vi "Update Slots.vi"(6 "FPGA Target":T1, 8 "error in (no error)":errorcluster, 10 "Scan Mode Slots":u32[](array[numeric]), 11 "Item Ref in":T2 format="%.0x") -> (0 "error out":errorcluster, 3 "Item Ref out":T2 format="%.0x")   [LabVIEW 2016, in "Scan Engine Custom Device.lvlib"]
uses:
  Scan Engine Custom Device.lvlib
  <vilib>/NI Veristand/Custom Device API/Custom Device API.lvlib
  Globals/Scan Engine GUIDs.vi
  Modules.lvlibp/RSI Module/Module Models.ctl
  <vilib>/NI Veristand/Custom Device API/Custom Device Item Ref.ctl
  Type Defs/FPGA Target.ctl
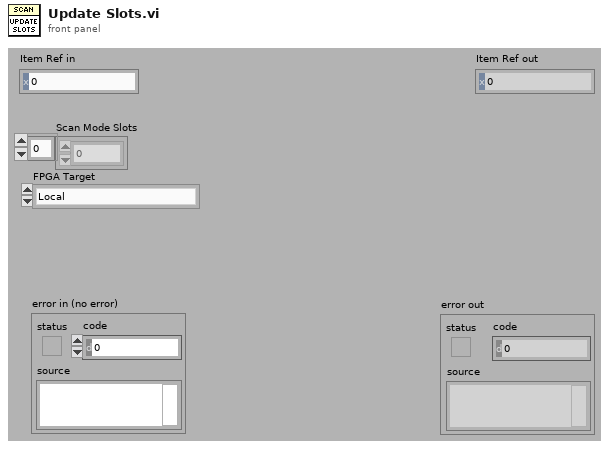
[diagram p1: front panel]
types:
  T1 = typedef "Scan Engine Custom Device.lvlib/FPGA Target.ctl" = enum16{"Local", "EtherCAT"}
  T2 = typedef "Custom Device API.lvlib/Custom Device Item Ref.ctl" = u64
  T3 = typedef "Modules.lvlibp/RSI Module.lvclass/Module Models.ctl" = enum16{"Empty", "NI 9201", "NI 9203", "NI 9205", "NI 9206", "NI 9207", "NI 9208", "NI 9211", "NI 9213", "NI 9214", "NI 9215", "NI 9217", "NI 9219", "NI 9221", "NI 9225", "NI 9227", "NI 9229", "NI 9233", "NI 9234", "NI 9235", "NI 9236", "NI 9237", "NI 9239", "NI 9263", "NI 9264", "NI 9265", "NI 9269", "NI 9375", "NI 9401", "NI 9402", "NI 9403", "NI 9411", "NI 9421", "NI 9422", "NI 9423", "NI 9425", "NI 9426", "NI 9435", "NI 9472", "NI 9474", "NI 9475", "NI 9476", "NI 9477", "NI 9478", "NI 9481", "NI 9482", "NI 9485"}
  T4 = typedef "Modules.lvlibp/Custom Device API.lvlib/Custom Device Item Ref.ctl" = u64
  T5 = typedef "Modules.lvlibp/RSI Module.lvclass/Slot Settings.ctl" = cluster{"Slot":u32, "EtherCAT?":bool}
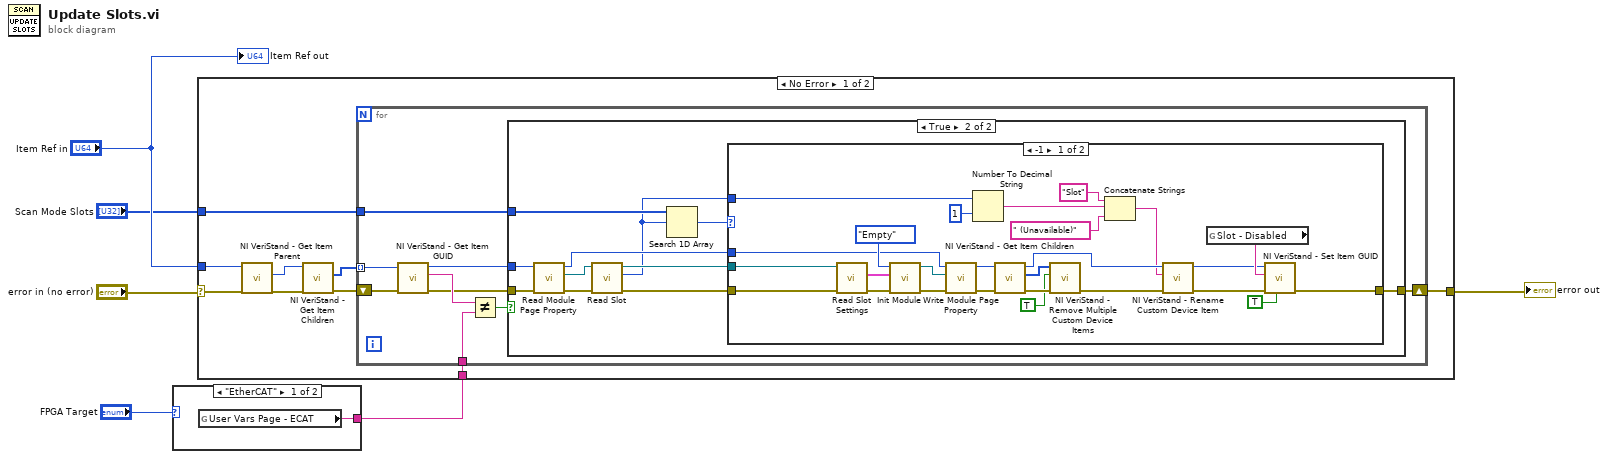
[diagram p0: block diagram]
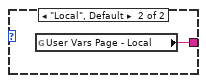
[diagram p2: hidden frame]
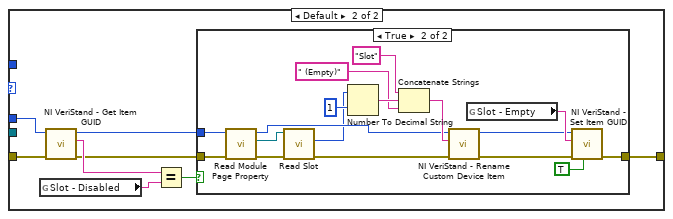
[diagram p4: hidden frame]
diagram:
  n1 = case shown="\"EtherCAT\"" "FPGA Target" {
    tunnel: [w7 w8] -> w1
    frame "EtherCAT" {
      n2 = global read "Scan Engine GUIDs.vi" "User Vars Page - ECAT"() -> (w7:string)
    }
    frame "Local", Default {
      n3 = global read "Scan Engine GUIDs.vi" "User Vars Page - Local"() -> (w8:string)
    }
  }
  n4 = case shown="No Error" "error in (no error)" {
    selector: "error in (no error)" -> [w16 w91]
    tunnel: [w9 w91] -> w5
    tunnel: "Item Ref in" -> [w17 _]
    tunnel: "Scan Mode Slots" -> [w11 _]
    tunnel: w1 -> [w10 _]
    frame No Error {
      n5 = call <vilib>:"NI VeriStand - Get Item Parent.vi"("error in (no error)"=w16, "Item Ref in"=w17) -> ("error out"=w15:errorcluster, "Parent Ref"=w14:T2)  [unwired: 6 in, 2 out]
      n6 = call <vilib>:"NI VeriStand - Get Item Children.vi"("error in (no error)"=w15, "Item Ref in"=w14) -> ("error out"=w13:errorcluster, "Child Refs"=w12:T2[])  [unwired: 6 in, 2 out]
      n7 = for {
        shift-right: [w18] -> w9
        shift-left: w13 -> [w26]
        tunnel: w12 -> [w25] mode=indexing
        tunnel: w11 -> [w19]
        tunnel: w10 -> [w24]
        n8 = call <vilib>:"NI VeriStand - Get Item GUID.vi"("error in (no error)"=w26, "Item Ref in"=w25) -> ("error out"=w21:errorcluster, "GUID"=w23:string, "Item Ref out"=w20:T2)  [unwired: 7 in]
        n9 = Not Equal?(x=w23, y=w24) -> (x != y?=w22:bool)
        n10 = case shown="True" w22 {
          tunnel: w21 -> [w27 w38]
          tunnel: w20 -> [_ w37]
          tunnel: w19 -> [_ w34]
          tunnel: [w27 w29] -> w18
          frame False {
          }
          frame True {
            n11 = call "Read Module Page Property.vi"("error in (no error)"=w38, "Node Ptr In"=w37) -> ("error out"=w36:errorcluster, "RSI Module"=w35:refnum<class "RSI Module.lvclass">, "Node Ptr Out"=w31:T4)  [unwired: 7 in]
            n12 = call "Read Slot.vi"("error in (no error)"=w36, "RSI Module in"=w35) -> ("error out"=w32:errorcluster, "Slot"=w28:u32, "RSI Module out"=w30:refnum<class "RSI Module.lvclass">)  [unwired: 7 in]
            n13 = Search 1D Array(1D array=w34, element=w28) -> (index of element=w33:i32)  [unwired: 1 in]
            n14 = case shown="-1" w33 {
              tunnel: w32 -> [w62 w67]
              tunnel: w31 -> [w56 w66]
              tunnel: w30 -> [w61 _]
              tunnel: [w49 w65] -> w29
              tunnel: w28 -> [w46 _]
              frame -1 {
                n15 = call "Read Slot Settings.vi"("error in (no error)"=w62, "RSI Module in"=w61) -> ("error out"=w60:errorcluster, "Slot Settings"=w59:T5)  [unwired: 7 in, 1 out]
                n16 = call "Init Module.vi"("error in (no error)"=w60, "Slot Settings"=w59, "Module Model"=Module_Models."Empty") -> ("error out"=w57:errorcluster, "RSI Module out"=w55:refnum<class "RSI Module.lvclass">)  [unwired: 7 in]
                n17 = call "Write Module Page Property.vi"("error in (no error)"=w57, "RSI Module"=w55, "Node Ptr In"=w56) -> ("error out"=w51:errorcluster, "Node Ptr Out"=w50:T4)  [unwired: 6 in, 1 out]
                n18 = Number To Decimal String(number=w46, width (-)=i16 1) -> (decimal integer string=w45:string)
                n19 = call <vilib>:"NI VeriStand - Get Item Children.vi"("error in (no error)"=w51, "Item Ref in"=w50) -> ("error out"=w54:errorcluster, "Child Refs"=w53:T2[], "Item Ref out"=w42:T2)  [unwired: 6 in, 1 out]
                n20 = call <vilib>:"NI VeriStand - Remove Multiple Custom Device Items.vi"("error in (no error)"=w54, "Force Delete (F)"=TRUE, "Item Refs in"=w53) -> ("error out"=w43:errorcluster)  [unwired: 7 in, 1 out]
                n21 = Concatenate Strings("Slot" ("string"), w45, " (Unavailable)" ("Section Name")) -> (w39:string)
                n22 = call <vilib>:"NI VeriStand - Rename Custom Device Item.vi"("error in (no error)"=w43, "New Name"=w39, "Item Ref in"=w42) -> ("error out"=w40:errorcluster, "Item Ref out"=w41:T2)  [unwired: 1 in, 6 out]
                n23 = global read "Scan Engine GUIDs.vi" "Slot - Disabled"() -> (w64:string)
                n24 = call <vilib>:"NI VeriStand - Set Item GUID.vi"("Refresh System Explorer Tree? (F)"=TRUE, "error in (no error)"=w40, "GUID"=w64, "Item Ref in"=w41) -> ("error out"=w49:errorcluster)  [unwired: 6 in, 1 out]
              }
              frame Default {
                n25 = global read "Scan Engine GUIDs.vi" "Slot - Disabled"() -> (w71:string)
                n26 = call <vilib>:"NI VeriStand - Get Item GUID.vi"("error in (no error)"=w67, "Item Ref in"=w66) -> ("error out"=w69:errorcluster, "GUID"=w72:string, "Item Ref out"=w68:T2)  [unwired: 7 in]
                n27 = Equal?(x=w72, y=w71) -> (x = y?=w70:bool)
                n28 = case shown="True" w70 {
                  tunnel: w69 -> [w73 w82]
                  tunnel: w68 -> [_ w83]
                  tunnel: [w73 w88] -> w65
                  frame False {
                  }
                  frame True {
                    n29 = call "Read Module Page Property.vi"("error in (no error)"=w82, "Node Ptr In"=w83) -> ("error out"=w85:errorcluster, "RSI Module"=w84:refnum<class "RSI Module.lvclass">, "Node Ptr Out"=w76:T4)  [unwired: 7 in]
                    n30 = call "Read Slot.vi"("error in (no error)"=w85, "RSI Module in"=w84) -> ("error out"=w74:errorcluster, "Slot"=w75:u32)  [unwired: 7 in, 1 out]
                    n31 = Number To Decimal String(number=w75, width (-)=i16 1) -> (decimal integer string=w80:string)
                    n32 = Concatenate Strings("Slot" ("string"), w80, " (Empty)" ("Section Name")) -> (w77:string)
                    n33 = call <vilib>:"NI VeriStand - Rename Custom Device Item.vi"("error in (no error)"=w74, "New Name"=w77, "Item Ref in"=w76) -> ("error out"=w87:errorcluster, "Item Ref out"=w86:T2)  [unwired: 1 in, 6 out]
                    n34 = global read "Scan Engine GUIDs.vi" "Slot - Empty"() -> (w89:string)
                    n35 = call <vilib>:"NI VeriStand - Set Item GUID.vi"("Refresh System Explorer Tree? (F)"=TRUE, "error in (no error)"=w87, "GUID"=w89, "Item Ref in"=w86) -> ("error out"=w88:errorcluster)  [unwired: 6 in, 1 out]
                  }
                }
              }
            }
          }
        }
      }
    }
    frame Error {
    }
  }
  "error out" <- w5
  "Item Ref out" <- "Item Ref in"
